vi "GetTdmConfig.vi"(3 "error in 2":errorcluster, 4 "String":string, 5 "storage refnum (file)":refnum<k20>) -> (0 "error in":errorcluster, 1 "Numeric":dbl, 2 "storage refnum (file) out":refnum<k20>)   [LabVIEW 2014]
uses:
  <vilib>/Platform/storage/lvStorage.llb/_queryPropPoly.vi
  <vilib>/Platform/storage/lvStorage.llb/_queryPropString.vi
  <vilib>/Platform/storage/lvStorage.llb/_queryGenericObjects.vi
  <vilib>/Platform/storage/lvStorage.llb/_loadAllDdt.vi
  <vilib>/Platform/storage/lvStorage.llb/xStorage/xStorageSupp/ErrorOut.vi
  <vilib>/Platform/storage/lvStorage.llb/xStorage/Read Data/Read Data.xnode
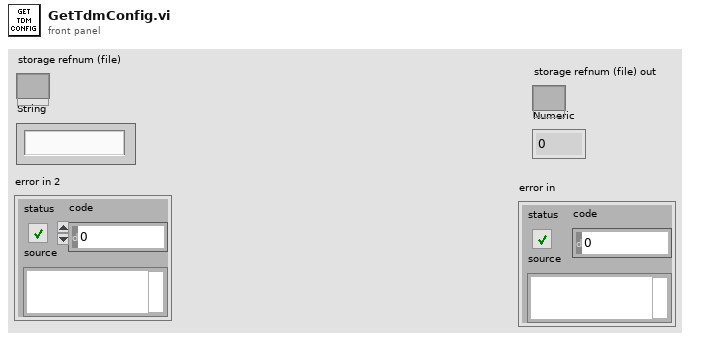
[diagram p1: front panel]
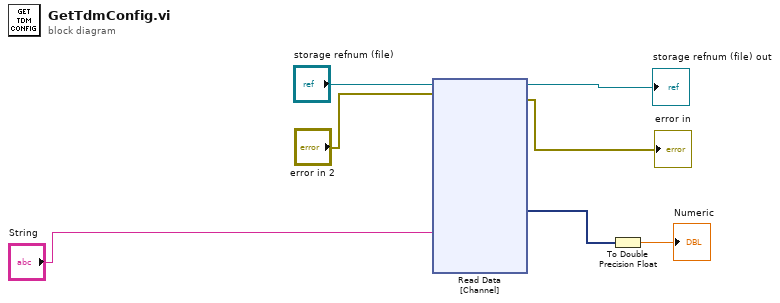
[diagram p0: block diagram]
diagram:
  n1 = xnode "Read Data\n[Channel]"("Name"="String", "storage refnum (file)"="storage refnum (file)", "error in"="error in 2") -> ("Signal"=w6:dynamicdata, "storage refnum (file) out"=→"storage refnum (file) out":refnum<k20>, "error out"=→"error in":errorcluster)  [unwired: 3 in, 1 out]
  n2 = To Double Precision Float(number=w6) -> (double precision float=→"Numeric":dbl)
